vi "1_DeepLTK_Boolean_Logic(Training).vi"() -> ()   [LabVIEW 2020]
uses:
  <vilib>/Ngene/DeepLTK/Toolkit/NN_Train/Controls/NN_Train_Params.ctl
  <vilib>/Ngene/DeepLTK/Toolkit/NN_Train/Controls/NN_Train_Optimizer.ctl
  <vilib>/Ngene/DeepLTK/Toolkit/NN_Train/Controls/NN_Train_Data_Sampling.ctl
  <vilib>/Ngene/DeepLTK/Toolkit/NN_Train/Controls/NN_LR_Policy_Cfg.ctl
  <vilib>/Ngene/DeepLTK/Toolkit/NN_Train/Controls/NN_LR_Policy_Type.ctl
  <vilib>/Ngene/DeepLTK/Toolkit/NN_Train/Controls/NN_Train_Session_Data.ctl
  <vilib>/Ngene/DeepLTK/Toolkit/NN_Layers/Layers/Input/Controls/NN_Layer_Config(Input1D).ctl
  <vilib>/Ngene/DeepLTK/Toolkit/NN_Network/Controls/NN_Save_Before_Destroy_Options.ctl
  <vilib>/Ngene/DeepLTK/Toolkit/NN_Data/API/DataSet_Types/NN_DataSet(In1D_Out1D).ctl
  <vilib>/Ngene/DeepLTK/Toolkit/NN_Data/API/DataRef_Types/NN_Data_ref(2D_SGL).ctl
  <vilib>/Ngene/DeepLTK/Toolkit/NN_Data/API/DataRef_Types/NN_Data_ref(1D_I32).ctl
  <vilib>/Ngene/DeepLTK/Toolkit/NN_Layers/Layers/FC/Controls/NN_Layer_Config(FC).ctl
  <vilib>/Ngene/DeepLTK/Toolkit/NN_Activations/Controls/NN_Activation_Type.ctl
  <vilib>/Ngene/DeepLTK/Toolkit/NN_Layers/Controls/NN_Layer_Init_Params.ctl
  <vilib>/Ngene/DeepLTK/Toolkit/NN_Layers/Controls/NN_Layer_Weight_Init_Type.ctl
  <vilib>/Ngene/DeepLTK/Toolkit/NN_Train/Loss_Functions/NN_Set_Loss(MSE).vi
  <vilib>/Ngene/DeepLTK/Toolkit/NN_Layers/Layers/FC/NN_Layer_Create(FC).vi
  <vilib>/Ngene/DeepLTK/Toolkit/NN_Layers/Layers/Input/NN_Layer_Create(Input1D).vi
  <vilib>/Ngene/DeepLTK/Toolkit/Deep_Learning_Toolkit_by_Ngene.lvlib
panel:
  out "Loss Value":sgl
  out "Session Data":T1
  out "Loss Chart":sgl(graph)=5.656097e-06
  in  "Stop Training":bool
  in  "LR_Decay_Params":T2={"Policy_Type"=enum."Step", "LR0"=10.0, "k"=10000.0, "WarmUp_Policy"=enum."Ramp", "WarmUp_Iter"=100, "WarmUp_Ratio"=10.0} {"WarmUp_Ratio" min=1; "WarmUp_Iter" min=1; "LR0" format="%.7f"}
  in  "NN_Train_Params":T4={"Optimizer"=enum."SGD", "Beta_1"=0.9, "Beta_2"=0.0, "Weight Decay(L1)"=1e-08, "Weight Decay(L2)"=1e-08, "Data_Sampling"=enum."Sequential"}
  # "Overview: Demonstrates the usage of DeepLTK (Deep Learning Toolkit for LabVIEW) for solving a Boolean Logic (AND) problem.\nRequirements: DeepLTK - Deep Learning Toolkit for LabVIEW (https://www.ngene.co/deep-learning-toolkit-for-labview)\nInstructions:\n1. Run the VI with default configurations.\n2. Observe how the training loss is decreasing.\n4. Press the Stop Train button when the \"Train Loss\" stops decreasing.\nMore Examples:  https://github.com/ngenehub/deepltk_examples"
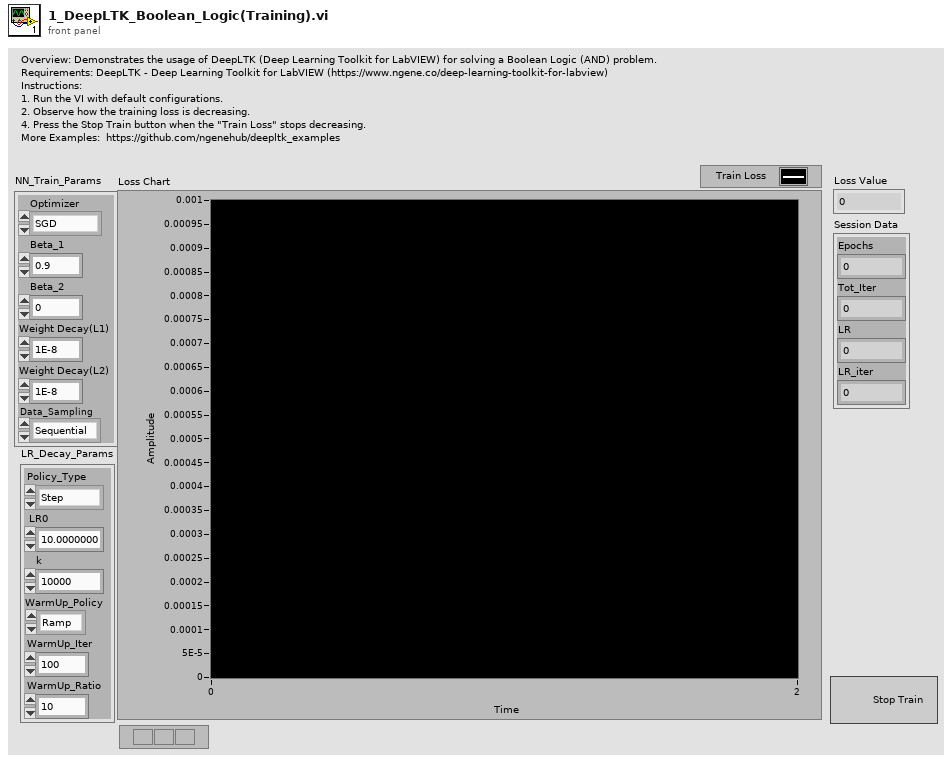
[diagram p1: front panel]
types:
  T1 = typedef "Deep_Learning_Toolkit_by_Ngene.lvlib/NN_Train_Session_Data.ctl" = cluster{"Epochs":sgl, "Tot_Iter":i32, "LR":sgl, "LR_iter":i32}
  T2 = typedef "Deep_Learning_Toolkit_by_Ngene.lvlib/NN_LR_Policy_Cfg.ctl" = cluster{"Policy_Type":T3, "LR0":dbl, "k":sgl, "WarmUp_Policy":enum16{"Step", "Ramp"}, "WarmUp_Iter":i32, "WarmUp_Ratio":sgl}
  T3 = typedef "Deep_Learning_Toolkit_by_Ngene.lvlib/NN_LR_Policy_Type.ctl" = enum16{"Manual", "Step", "Exp", "1/t"}
  T4 = typedef "Deep_Learning_Toolkit_by_Ngene.lvlib/NN_Train_Params.ctl" = cluster{"Optimizer":T5, "Beta_1":sgl, "Beta_2":sgl, "Weight Decay(L1)":sgl, "Weight Decay(L2)":sgl, "Data_Sampling":T6}
  T5 = typedef "Deep_Learning_Toolkit_by_Ngene.lvlib/NN_Train_Optimizer.ctl" = enum16{"SGD", "Adam", "Adagrad", "Adadelta", "RMSProp", "Nesterov"}
  T6 = typedef "Deep_Learning_Toolkit_by_Ngene.lvlib/NN_Train_Data_Sampling.ctl" = enum16{"Random", "Sequential"}
  T7 = typedef "Deep_Learning_Toolkit_by_Ngene.lvlib/NN_Layer_Config(FC).ctl" = cluster{"Name":string, "Size":i32, "BN":bool, "Activation":T8, "Init_Params":T9, "Custom_Params":string}
  T8 = typedef "Deep_Learning_Toolkit_by_Ngene.lvlib/NN_Activation_Type.ctl" = enum16{"Sigmoid", "ReLU", "LReLU", "ReLU6", "tanh", "Swish", "Mish", "None"}
  T9 = typedef "Deep_Learning_Toolkit_by_Ngene.lvlib/NN_Layer_Init_Params.ctl" = cluster{"Init_Type":T10, "Value":sgl}
  T10 = typedef "Deep_Learning_Toolkit_by_Ngene.lvlib/NN_Layer_Weight_Init_Type.ctl" = enum16{"Const", "Uniform", "Gaussian", "Xavier"}
  T11 = typedef "Deep_Learning_Toolkit_by_Ngene.lvlib/NN_DataSet(In1D_Out1D).ctl" = cluster{"Inputs Ref.":T12, "Outputs Ref.":T12, "Dims_In":i32, "Dataset_Size":i32, "Outputs_idx Ref.":T13, "Dims_Out":i32, "Labels":string[], "File Paths":path[]}
  T12 = typedef "Deep_Learning_Toolkit_by_Ngene.lvlib/NN_Data_ref(2D_SGL).ctl" = refnum<data-value>
  T13 = typedef "Deep_Learning_Toolkit_by_Ngene.lvlib/NN_Data_ref(1D_I32).ctl" = refnum<data-value>
  T14 = typedef "Deep_Learning_Toolkit_by_Ngene.lvlib/NN_Save_Before_Destroy_Options.ctl" = cluster{"CFG?":bool, "Weights?":bool, "Render?":bool}
  T15 = typedef "Deep_Learning_Toolkit_by_Ngene.lvlib/NN_Layer_Config(Input1D).ctl" = cluster{"Name":string, "Size":i32}
  T16 = typedef "Deep_Learning_Toolkit_by_Ngene.lvlib/NN.ctl" = cluster{"Name":string, "No of Layers":i32, "mBatch":i32, "Layers":T17[], "Dimty":T18, "Dims_In":T19, "Dims_Out":T19, "Working_Dir":path, "Train?":bool, "Train_Params":T4, "LR_Update_Policy":T2, "Session Data":T1, "Ground_truth":T20, "NNg_hdls":T21, "NN_Device":T22, "GPU Id":i32, "Labels":string[], "Receptive Field":T23[], "Loss_Type":T24, "Loss_Cfg_Prms":variant}
  T17 = typedef "Deep_Learning_Toolkit_by_Ngene.lvlib/NN_Layer_ref.ctl" = refnum<data-value>
  T18 = typedef "Deep_Learning_Toolkit_by_Ngene.lvlib/NN_In_Out_Dim-ty.ctl" = enum8{"In1D_Out1D", "In3D_Out1D", "In3D_Out3D", "In3D_OutBBox"}
  T19 = typedef "Deep_Learning_Toolkit_by_Ngene.lvlib/NN_Dims(C,H,W).ctl" = cluster{"C":i32, "H":i32, "W":i32}
  T20 = typedef "Deep_Learning_Toolkit_by_Ngene.lvlib/NN_Ground_truth.ctl" = cluster{"Y":variant, "Y_idx":T13}
  T21 = typedef "Deep_Learning_Toolkit_by_Ngene.lvlib/nng_cuda_handles.ctl" = cluster{"cudnn":u64, "cublas":u64, "stream":u64, "curand":u64}
  T22 = typedef "Deep_Learning_Toolkit_by_Ngene.lvlib/NN_Device.ctl" = enum16{"CPU", "GPU"}
  T23 = typedef "Deep_Learning_Toolkit_by_Ngene.lvlib/NN_Dims(V,H).ctl" = cluster{"V":i32, "H":i32}
  T24 = typedef "Deep_Learning_Toolkit_by_Ngene.lvlib/NN_Loss_Type.ctl" = enum16{"None", "MSE", "CrossEntropy", "YOLO_v2"}
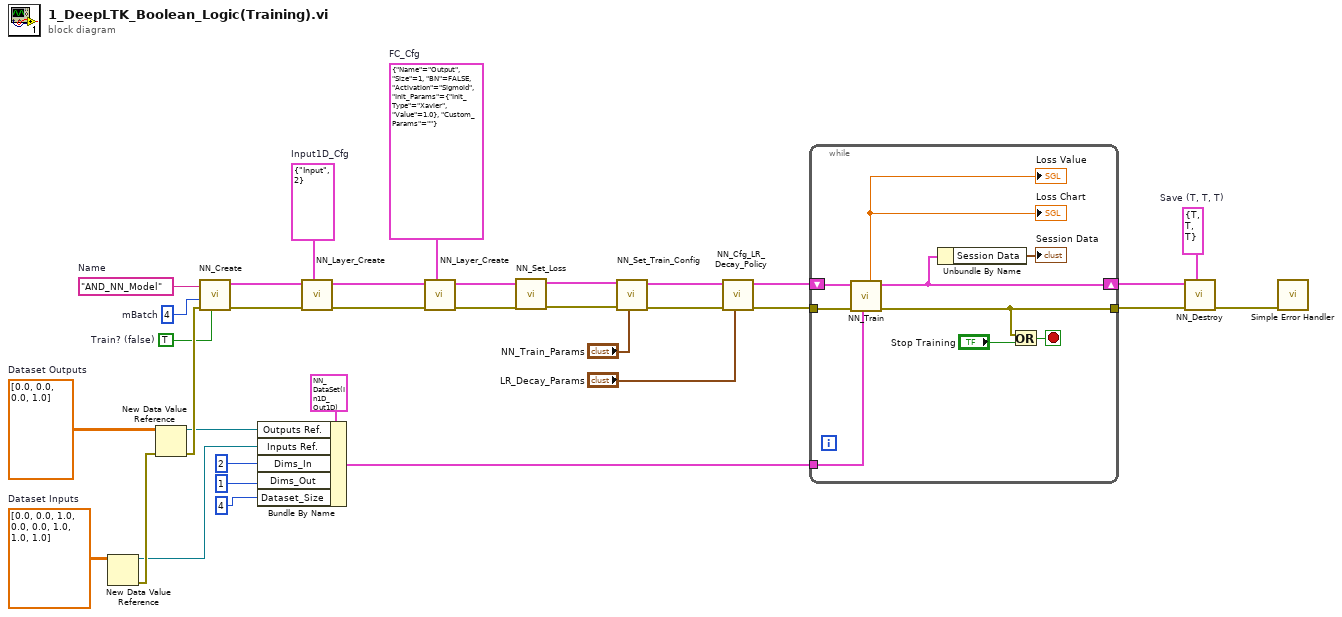
[diagram p0: block diagram]
diagram:
  w3 = T7 {"Name"="Output", "Size"=1, "BN"=FALSE, "Activation"=enum."Sigmoid", "Init_Params"={"Init_Type"=enum."Xavier", "Value"=1.0}, "Custom_Params"=""}  # FC_Cfg
  w5 = T14 {"CFG?"=TRUE, "Weights?"=TRUE, "Render?"=TRUE}  # Save (T, T, T)
  w17 = 4  # mBatch
  w22 = T15 {"Name"="Input", "Size"=2}  # Input1D_Cfg
  w23 = "AND_NN_Model"  # Name
  w24 = TRUE  # Train? (false)
  w30 = sgl[][] [[0.0], [0.0], [0.0], [1.0]]  # Dataset Outputs
  w31 = sgl[][] [[0.0, 0.0], [1.0, 0.0], [0.0, 1.0], [1.0, 1.0]]  # Dataset Inputs
  n1 = New Data Value Reference(data value=w31) -> (data value reference=w29:refnum<data-value>, error out=w34:errorcluster)  [unwired: 1 in]
  n2 = New Data Value Reference(data value=w30, error in=w34) -> (data value reference=w28:refnum<data-value>, error out=w33:errorcluster)
  n3 = call <vilib>:"NN_Create.vi"("Train? (false)"=w24, "error in (no error)"=w33, "mBatch (1)"=w17, "Name"=w23) -> ("error out"=w14:errorcluster, "NN out"=w16:T16)  [unwired: 6 in]
  n4 = Bundle By Name(cluster=T11 {"Inputs Ref."=refnum, "Outputs Ref."=refnum, "Dims_In"=0, "Dataset_Size"=0, "Outputs_idx Ref."=refnum, "Dims_Out"=0, "Labels"=[], "File Paths"=[]} ("Dataset(In1D_Out1D)"), "Outputs Ref."=w28, "Inputs Ref."=w29, "Dims_In"=2, "Dims_Out"=1, "Dataset_Size"=4) -> (w9:T11)
  n5 = call-poly <vilib>:"NN_Layer_Create.vi"("Input1D_Cfg"=w22, "error in (no error)"=w14, "NN in"=w16) -> ("error out"=w13:errorcluster, "NN out"=w15:T16)  [unwired: 6 in, 1 out]
  n6 = call-poly <vilib>:"NN_Layer_Create.vi"("FC_Cfg"=w3, "error in (no error)"=w13, "NN in"=w15) -> ("error out"=w1:errorcluster, "NN out"=w2:T16)  [unwired: 6 in, 1 out]
  n7 = call-poly <vilib>:"NN_Set_Loss.vi"("error in (no error)"=w1, "NN in"=w2) -> ("error out"=w6:errorcluster, "NN out"=w7:T16)  [unwired: 8 in]
  n8 = call <vilib>:"NN_Set_Train_Config.vi"("NN_Train_Params"="NN_Train_Params", "error in (no error)"=w6, "NN in"=w7) -> ("error out"=w19:errorcluster, "NN out"=w18:T16)  [unwired: 7 in]
  n9 = call <vilib>:"NN_Cfg_LR_Decay_Policy.vi"("LR_Decay_Params"="LR_Decay_Params", "error in (no error)"=w19, "NN in"=w18) -> ("error out"=w8:errorcluster, "NN out"=w10:T16)  [unwired: 7 in]
  n10 = while {
    shift-right: [w43] -> w12
    shift-left: w10 -> [w41]
    tunnel: [w35] -> w11
    tunnel: w8 -> [w39]
    tunnel: w9 -> [w38]
    stop <- w36 stop-if-true
    n11 = call <vilib>:"NN_Train.vi"("Train Dataset"=w38, "error in (no error)"=w39, "NN in"=w41) -> ("error out"=w35:errorcluster, "NN out"=w43:T16, "Loss"=→"Loss Chart" →"Loss Value":sgl)  [unwired: 5 in, 1 out]
    n12 = Unbundle By Name(w43) -> ("Session Data"=→"Session Data":T1)
    n13 = Or(x=w35, y="Stop Training") -> (x .or. y?=w36:bool)
  }
  n14 = call <vilib>:"NN_Destroy.vi"("Save (T, T, T)"=w5, "error in (no error)"=w11, "NN in"=w12) -> ("error out"=w4:errorcluster)  [unwired: 8 in]
  n15 = call <vilib>:"Simple Error Handler.vi"("error in (no error)"=w4) -> ()  [unwired: 4 in, 5 out]
